vi "Read Actual Values From Log File.vi"(8 "Error In":errorcluster, 9 "Signal":string, 10 "Log":path, 11 "Test Data":T1[](array[typedef])) -> (0 "Error Out":errorcluster, 1 "System Time":dbl[](array[numeric]), 2 "Actual Values":dbl[](array[numeric]), 3 "Idx":i32)   [LabVIEW 2011]
uses:
  Controls/Test Column Data.ctl
  Channel path to TDMS Group and Channel.vi
  Find Index of Timestamps.vi
  <vilib>/Utility/error.llb/Error Cluster From Error Code.vi
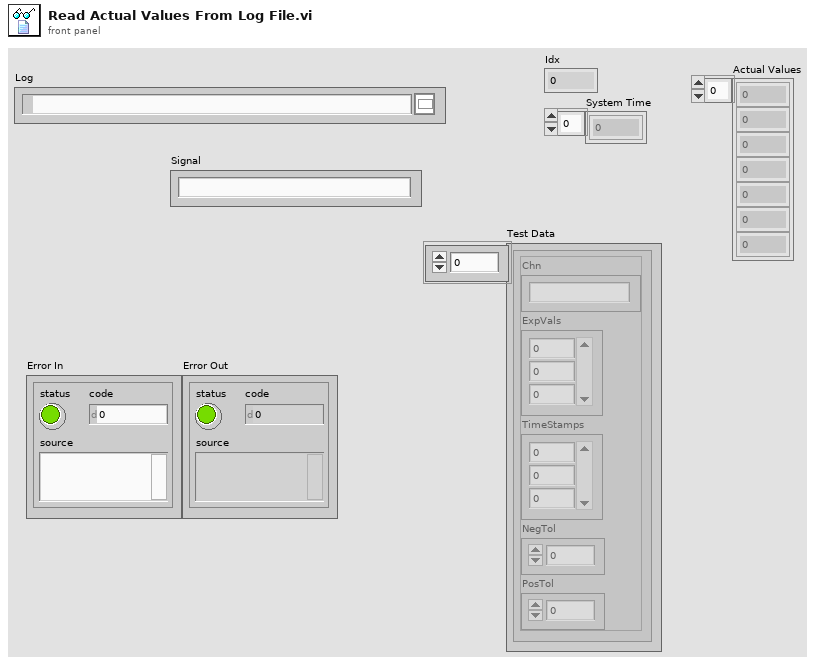
[diagram p1: front panel]
types:
  T1 = typedef "Test Column Data.ctl" = cluster{"Chn":string, "ExpVals":dbl[], "TimeStamps":i64[], "NegTol":dbl, "PosTol":dbl}
  T2 = enum16{"open", "open or create", "create or replace", "create", "open (read-only)"}
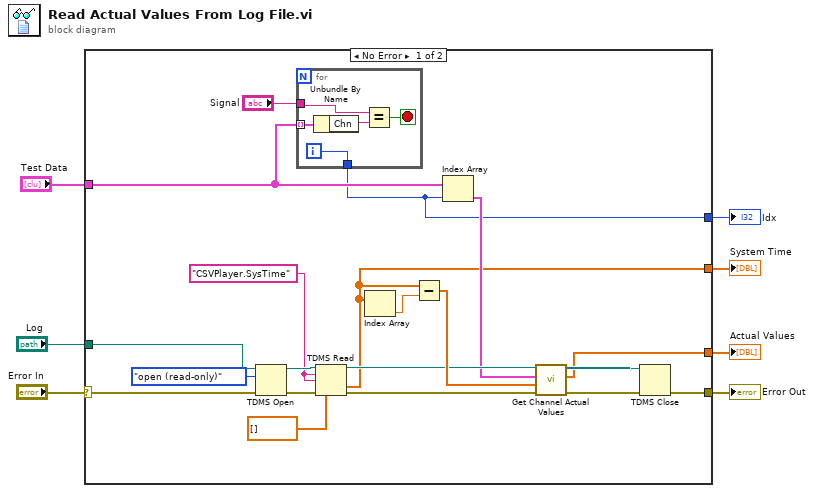
[diagram p0: block diagram]
diagram:
  n1 = case shown="No Error" "Error In" {
    selector: "Error In" -> [w15 w33]
    tunnel: "Log" -> [w27 _]
    tunnel: "Test Data" -> [w12 _]
    tunnel: [w16 w33] -> w6
    tunnel: [w11 _] -> w3
    tunnel: [w10 _] -> w2
    tunnel: [w9 _] -> w1
    frame No Error {
      w24 = "CSVPlayer.SysTime" ("group name in")
      n2 = TDMS Open(8:w15, 10:T2."open (read-only)" ("operation (0:open)"), 11:w27) -> (0:w26:errorcluster, 3:w25:refnum<k34>)  [unwired: 3 in]
      n3 = for {
        tunnel: w12 -> [w32] mode=indexing
        tunnel: "Signal" -> [w30]
        tunnel: [w28] -> w9
        i -> [w28]
        stop <- w29 stop-if-true
        n4 = Unbundle By Name(w32) -> ("Chn"=w31:string)
        n5 = Equal?(x=w30, y=w31) -> (x = y?=w29:bool)
      }
      n6 = TDMS Read(0:w25, 5:w24, 7:w24, 11:w26, 12:dbl[] []) -> (4:w20:refnum<k34>, 10:w10:dbl[], 15:w21:errorcluster)  [unwired: 3 in, 3 out]
      n7 = Index Array(array=w10) -> (element=w23:dbl)  [unwired: 1 in]
      n8 = Subtract(x=w10, y=w23) -> (x-y=w22:dbl[])
      n9 = Index Array(array=w12, index=w9) -> (element=w13:T1)
      n10 = call "Get Channel Actual Values.vi"("error in (no error)"=w21, "System Time"=w22, "Column Data"=w13, "TDMS in"=w20) -> ("error out"=w18:errorcluster, "Actual Values"=w11:dbl[], "TDMS Out"=w17:refnum<k34>)  [unwired: 5 in]
      n11 = TDMS Close(8:w18, 11:w17) -> (0:w16:errorcluster)  [unwired: 1 out]
    }
    frame Error {
    }
  }
  "Error Out" <- w6
  "Actual Values" <- w3
  "System Time" <- w2
  "Idx" <- w1
